vi "Run.vi"(8 "error in (no error)":errorcluster, 11 "JSON Lexer in":refnum<class "JSON Lexer.lvclass">) -> (0 "error out":errorcluster, 3 "JSON Lexer out":refnum<class "JSON Lexer.lvclass">)   [LabVIEW 2019, in "JKI JSON Serialization.lvlib" / "JSON Lexer.lvclass"]
doc: "JKI JSON 1.1.10.37\nTomi Maila - JKI\nCopyright (c) 2017, JKI"
uses:
  JSON Lexer.lvclass
  JSON Lexer States.ctl
  JSON Lexer.lvclass/JSON Lexer.ctl
  Unicode/UTF-8 String/UTF-8 String.lvclass/UTF-8 String.ctl
  Backup.vi
  Next.vi
  Unicode/UTF-8 String/Index Rune as UTF-8 Substring.vi
  Ignore.vi
  Unicode/UTF-8 String/Next Rune As UTF-8 Substring.vi
  Unicode/UTF-8 String/Bytes In Rune.vi
  Emit.vi
  Accept.vi
  Accept Multiple.vi
  Match.vi
  Peek.vi
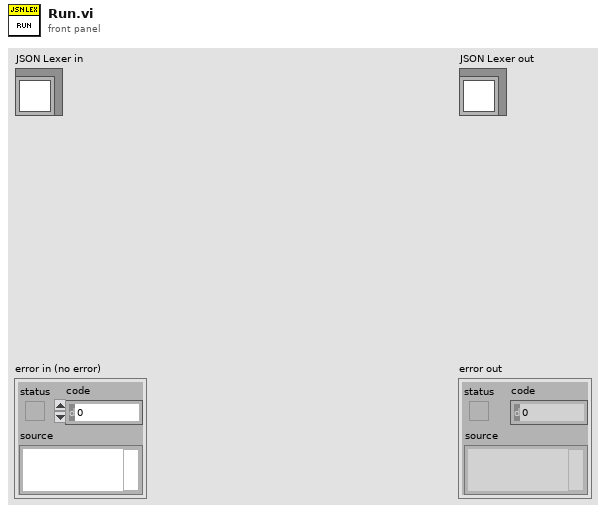
[diagram p1: front panel]
types:
  T1 = typedef "JKI JSON Serialization.lvlib/JSON Lexer.lvclass/JSON Lexer States.ctl" = enum16{"Undefined", "Value", "String", "Numeric", "Number", "Symbol", "Symbolic Number"}
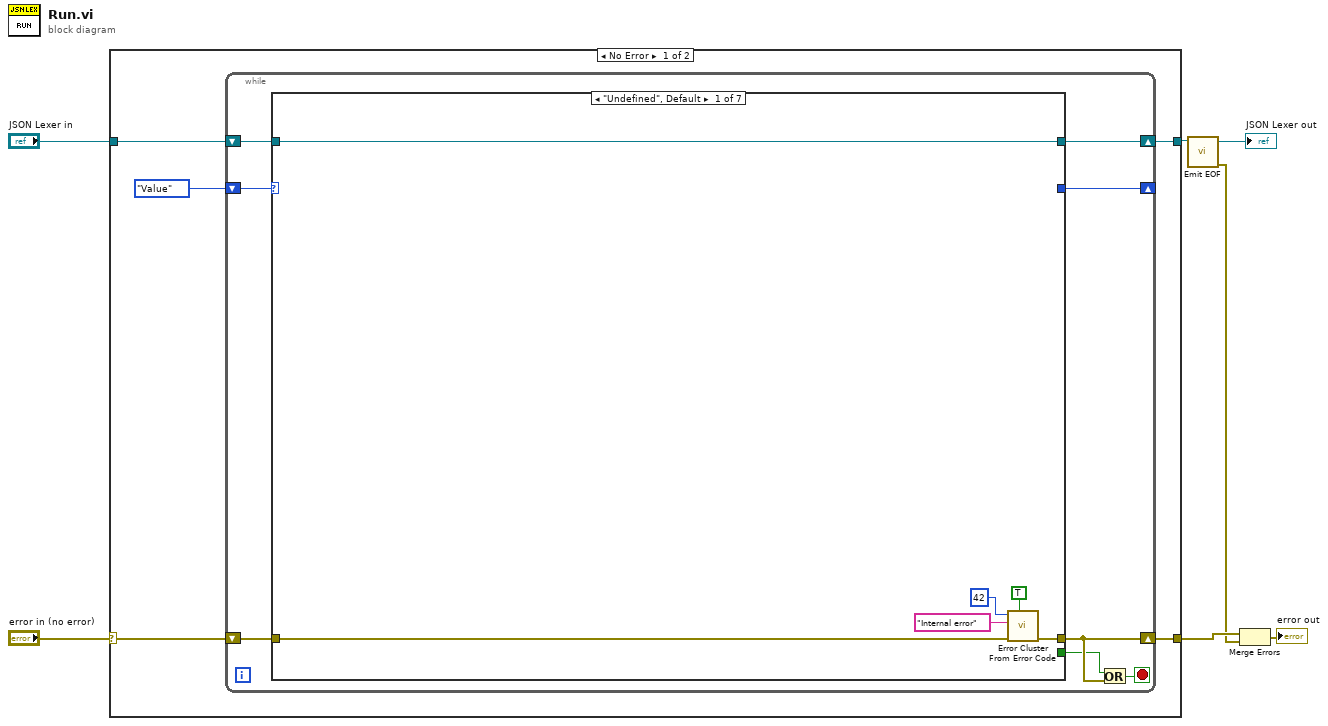
[diagram p0: block diagram]
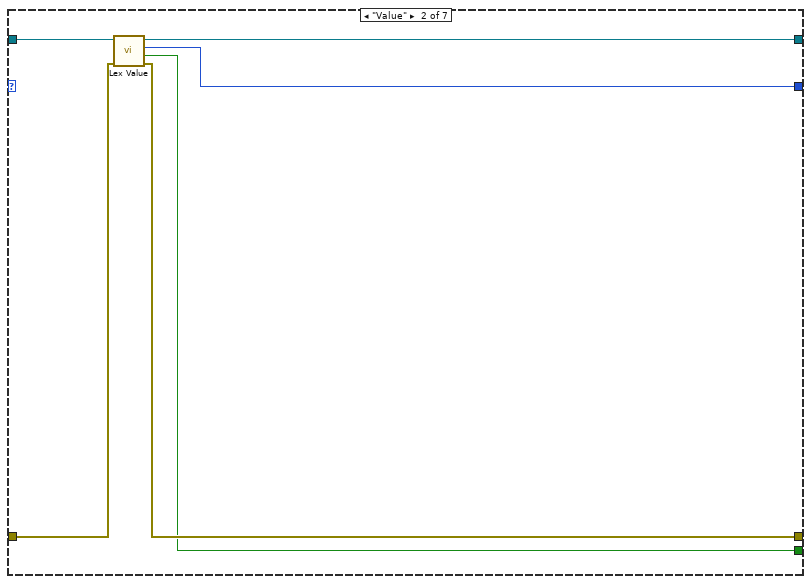
[diagram p2: hidden frame]
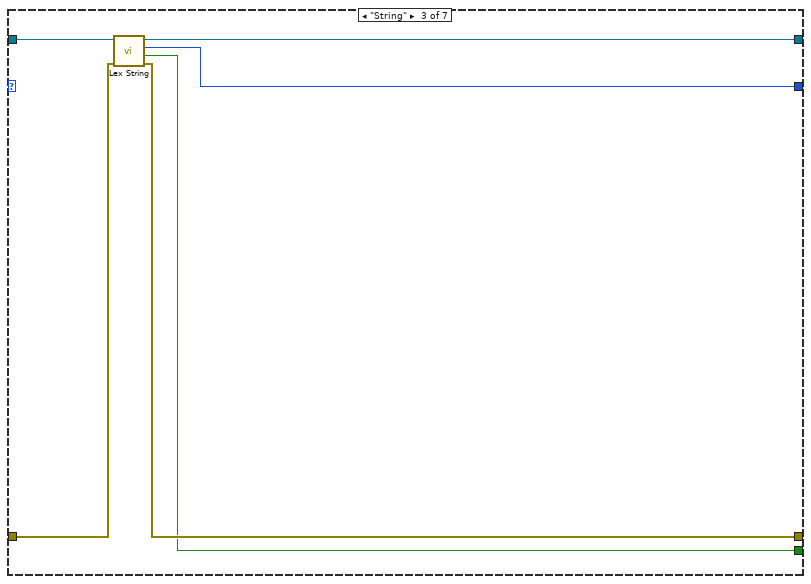
[diagram p3: hidden frame]
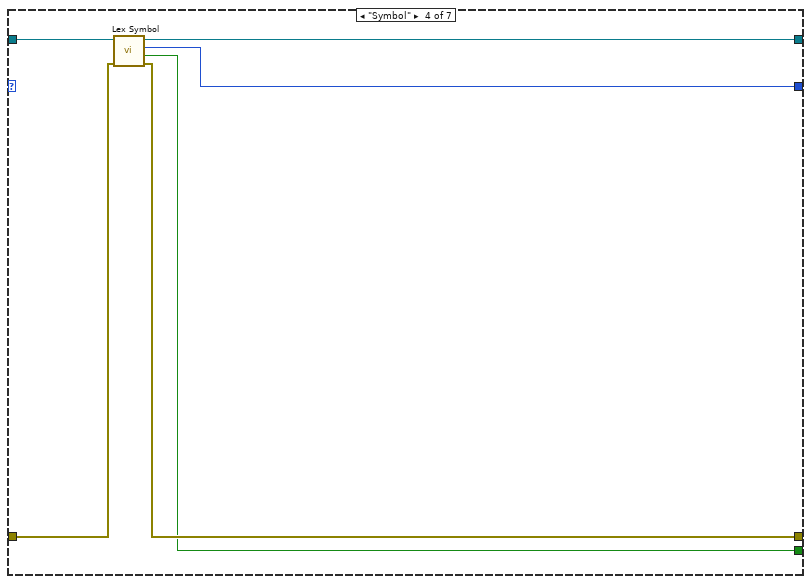
[diagram p4: hidden frame]
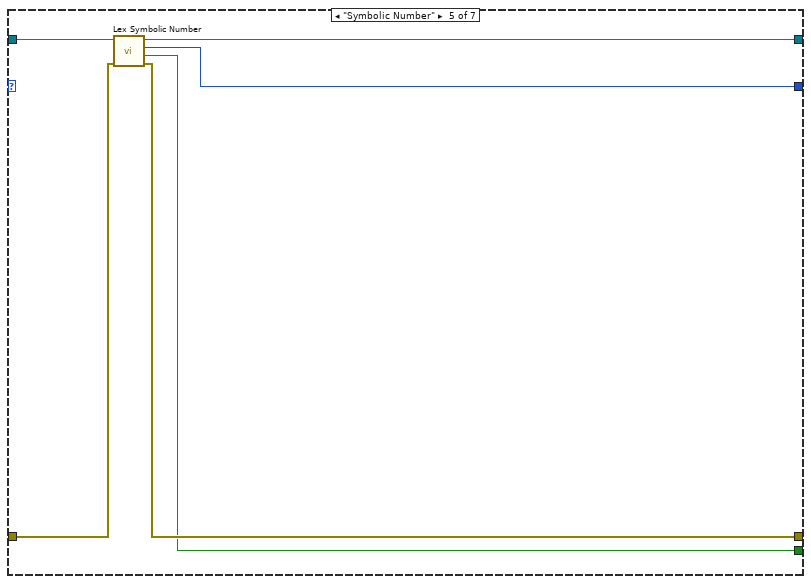
[diagram p5: hidden frame]
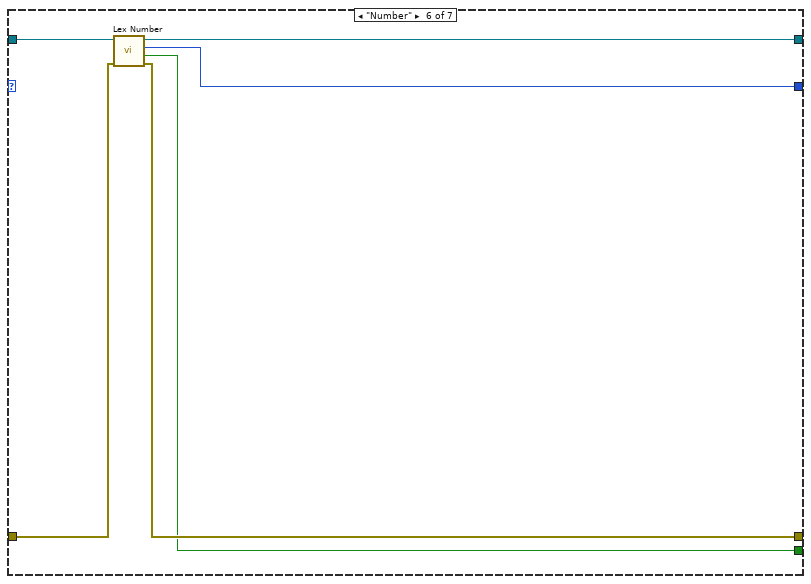
[diagram p6: hidden frame]
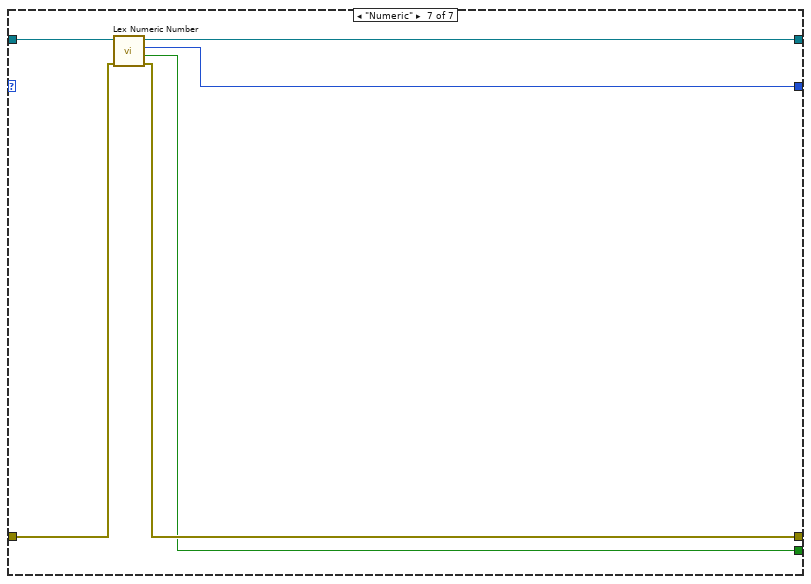
[diagram p7: hidden frame]
diagram:
  n1 = case shown="No Error" "error in (no error)" {
    selector: "error in (no error)" -> [w11 w64]
    tunnel: [w8 w64] -> w3
    tunnel: [w9 w63] -> w5
    tunnel: "JSON Lexer in" -> [w12 w63]
    frame No Error {
      n2 = while {
        shift-right: [w19] -> w9
        shift-left: w12 -> [w20]
        shift-right: [w16] -> w8
        shift-left: w11 -> [w18]
        shift-right: [w15] -> _
        shift-left: JSON_Lexer_States."Value" ("JSON Lexer State") -> [w14]
        stop <- w17 stop-if-true
        n3 = case shown="\"Undefined\", Default" w14 {
          tunnel: w20 -> [w26 w32 w38 w44 w50 w56 w62]
          tunnel: [w26 w31 w37 w43 w49 w55 w61] -> w19
          tunnel: w18 -> [w24 w30 w36 w42 w48 w54 w60]
          tunnel: [w25 w29 w35 w41 w47 w53 w59] -> w16
          tunnel: [_ w28 w34 w40 w46 w52 w58] -> w15
          tunnel: [_ w27 w33 w39 w45 w51 w57] -> w13
          frame "Undefined", Default {
            n4 = call <vilib>:"Error Cluster From Error Code.vi"("show call chain? (False)"=TRUE, "error in (no error)"=w24, "error message (\"\")"="Internal error" ("error message (\"\")"), "error code (0)"=42) -> ("error out"=w25:errorcluster)  [unwired: 5 in]
          }
          frame "Value" {
            n5 = call "Lex Value.vi"("error in (no error)"=w30, "JSON Lexer in"=w32) -> ("error out"=w29:errorcluster, "EOF"=w27:bool, "Next State"=w28:T1, "JSON Lexer out"=w31:refnum<class "JSON Lexer.lvclass">)  [unwired: 6 in]
          }
          frame "String" {
            n6 = call "Lex String.vi"("error in (no error)"=w36, "JSON Lexer in"=w38) -> ("error out"=w35:errorcluster, "EOF"=w33:bool, "Next State"=w34:T1, "JSON Lexer out"=w37:refnum<class "JSON Lexer.lvclass">)  [unwired: 6 in]
          }
          frame "Symbol" {
            n7 = call "Lex Symbol.vi"("error in (no error)"=w42, "JSON Lexer in"=w44) -> ("error out"=w41:errorcluster, "EOF"=w39:bool, "Next State"=w40:T1, "JSON Lexer out"=w43:refnum<class "JSON Lexer.lvclass">)  [unwired: 6 in]
          }
          frame "Symbolic Number" {
            n8 = call "Lex Symbolic Number.vi"("error in (no error)"=w48, "JSON Lexer in"=w50) -> ("error out"=w47:errorcluster, "EOF"=w45:bool, "Next State"=w46:T1, "JSON Lexer out"=w49:refnum<class "JSON Lexer.lvclass">)  [unwired: 6 in]
          }
          frame "Number" {
            n9 = call "Lex Number.vi"("error in (no error)"=w54, "JSON Lexer in"=w56) -> ("error out"=w53:errorcluster, "EOF"=w51:bool, "Next State"=w52:T1, "JSON Lexer out"=w55:refnum<class "JSON Lexer.lvclass">)  [unwired: 6 in]
          }
          frame "Numeric" {
            n10 = call "Lex Numeric Number.vi"("error in (no error)"=w60, "JSON Lexer in"=w62) -> ("error out"=w59:errorcluster, "EOF"=w57:bool, "Next State"=w58:T1, "JSON Lexer out"=w61:refnum<class "JSON Lexer.lvclass">)  [unwired: 6 in]
          }
        }
        n11 = Or(x=w13, y=w16) -> (x .or. y?=w17:bool)
      }
    }
    frame Error {
    }
  }
  n12 = call "Emit EOF.vi"("JSON Lexer in"=w5) -> ("error out"=w1:errorcluster, "JSON Lexer out"=→"JSON Lexer out":refnum<class "JSON Lexer.lvclass">)  [unwired: 9 in]
  n13 = Merge Errors(w3, w1) -> (→"error out":errorcluster)
